vi "DUAL GAUGE-RW Sensor On-Off.vi"(0 "Referenz in":refnum<visa-resource-name>, 1 "W/R":bool, 5 "No ON/OFF ID´s":string[](array[string])=["noSe", "LIN", "PIR", "CO9"], 7 "Sensor 1 Set":u8(ring) items=["no change / no sensor", "off", "automatic", "on"], 9 "Sensor 2 Set":u8(ring) items=["no change / no sensor", "off", "automatic", "on"], 11 "Fehler (Eingang)":errorcluster) -> (4 "Referenz out":refnum<visa-resource-name>, 8 "Sensor 1 Set":u8(ring) items=["no change / no sensor", "off", "automatic", "on"], 10 "Sensor 2 Set":u8(ring) items=["no change / no sensor", "off", "automatic", "on"], 15 "Cluster (Ausgang)":errorcluster)   [LabVIEW 2017, in "Dual Gauge.lvlib"]
uses:
  <userlib>/Dual Gauge/Dual Gauge.lvlib
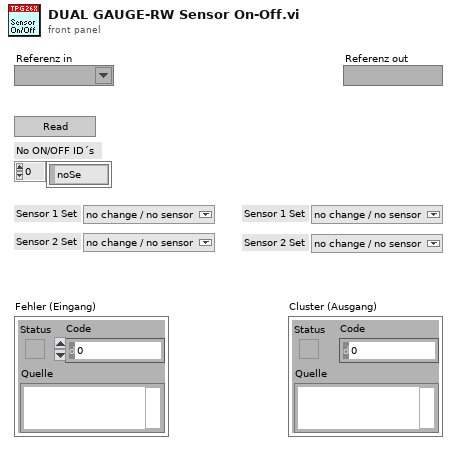
[diagram p1: front panel]
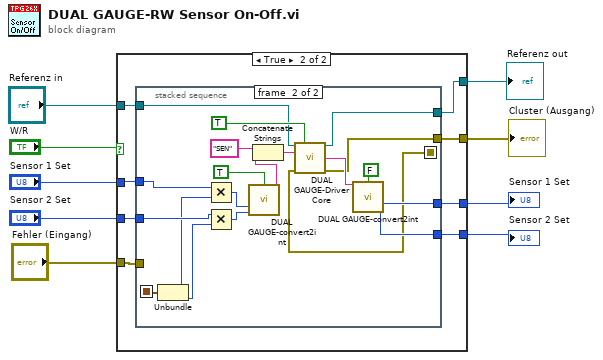
[diagram p0: block diagram]
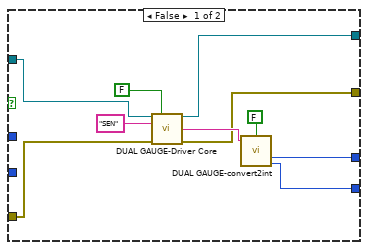
[diagram p2: hidden frame]
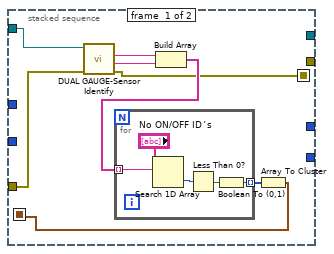
[diagram p3: hidden frame]
diagram:
  n1 = case shown="True" "W/R" {
    tunnel: "Sensor 1 Set" -> [_ w24]
    tunnel: "Sensor 2 Set" -> [_ w23]
    tunnel: [w18 w27] -> w4
    tunnel: [w17 w25] -> w5
    tunnel: [w16 w26] -> w6
    tunnel: [w12 w22] -> w3
    tunnel: "Referenz in" -> [w11 w21]
    tunnel: "Fehler (Eingang)" -> [w10 w20]
    frame False {
      n2 = call <userlib>:"DUAL GAUGE-Driver Core.vi"("Referenz in"=w11, "Write/Read"=FALSE, "Command"="SEN", "Fehler (Eingang)"=w10) -> ("Referenz out"=w12:refnum<visa-resource-name>, "String Out"=w19:string, "Cluster (Ausgang)"=w18:errorcluster)  [unwired: 9 in]
      n3 = call <userlib>:"DUAL GAUGE-convert2int.vi"("String in"=w19, "W/R [W: Int in; Str out ]"=FALSE) -> ("Integer3 out"=w16:u8, "Integer4 out"=w17:u8)  [unwired: 9 in, 3 out]
    }
    frame True {
      n4 = stacked-sequence {
        seq-local: [w33 _] -> [_ w55]
        seq-local: [w28 _] -> [_ w41]
        tunnel: [_ w58] -> w27
        tunnel: [_ w57] -> w26
        tunnel: [_ w56] -> w25
        tunnel: w24 -> [_ w50]
        tunnel: w23 -> [_ w49]
        tunnel: [_ w43] -> w22
        tunnel: w21 -> [w32 w42]
        tunnel: w20 -> [w29 _]
        frame #0 {
          n5 = call <userlib>:"DUAL GAUGE-Sensor Identify.vi"("Fehler (Eingang)"=w29, "Referenz in"=w32) -> ("Cluster (Ausgang)"=w28:errorcluster, "Sensor 2"=w30:string, "Sensor 1"=w31:string)  [unwired: 6 in, 1 out]
          n6 = Build Array(w31, w30) -> (w35:string[])
          n7 = for {
            tunnel: [w38] -> w34 mode=indexing
            tunnel: w35 -> [w36] mode=indexing
            n8 = Search 1D Array(1D array="No ON/OFF ID´s", element=w36) -> (index of element=w40:i32)  [unwired: 1 in]
            n9 = Less Than 0?(x=w40) -> (x < 0?=w39:bool)
            n10 = Boolean To (0,1)(Boolean=w39) -> (0, 1=w38:i16)
          }
          n11 = Array To Cluster(array=w34) -> (cluster=w33:cluster{"[0]":i16, "[1]":i16})
        }
        frame #1 {
          n12 = Unbundle(w55) -> ("[0]"=w48:i16, "[1]"=w47:i16)
          n13 = Multiply(x=w50, y=w48) -> (x*y=w52:i16)
          n14 = Multiply(x=w49, y=w47) -> (x*y=w51:i16)
          n15 = call <userlib>:"DUAL GAUGE-convert2int.vi"("W/R [W: Int in; Str out ]"=TRUE, "Integer1 in"=w52, "Integer2 in"=w51) -> ("String out"=w46:string)  [unwired: 8 in, 4 out]
          n16 = Concatenate Strings("SEN", w46) -> (w44:string)
          n17 = call <userlib>:"DUAL GAUGE-Driver Core.vi"("Referenz in"=w42, "Write/Read"=TRUE, "Command"=w44, "Fehler (Eingang)"=w41) -> ("Referenz out"=w43:refnum<visa-resource-name>, "String Out"=w60:string, "Cluster (Ausgang)"=w58:errorcluster)  [unwired: 9 in]
          n18 = call <userlib>:"DUAL GAUGE-convert2int.vi"("String in"=w60, "W/R [W: Int in; Str out ]"=FALSE) -> ("Integer3 out"=w57:u8, "Integer4 out"=w56:u8)  [unwired: 9 in, 3 out]
        }
      }
    }
  }
  "Sensor 2 Set" <- w5
  "Sensor 1 Set" <- w6
  "Cluster (Ausgang)" <- w4
  "Referenz out" <- w3
